vi "generate_DAC_voltages.vi"(8 "derived values":T1, 9 "scan specification":T4={"x amplitude"=0, "x resolution (pixels)"=0, "x offset fly-forward (iterations)"=0, "x offset fly-back (iterations)"=0, "y resolution (nr. of lines)"=0, "y step size"=0, "iterations per pixel"=0, "number of frames"=0, "y offset (pixels)"=0, "number of y-brake lines  (before y-fly-back)"=0, "number y-brake lines (after y-fly-back)"=0, "number of y-fly-back steps"=8, "lines per z step"=0, "number of z/intensity tuples"=0}, 10 "counter cluster in":T2, 11 "resonant trigger":bool) -> (0 "acquire?":bool, 1 "fly-back acquisition phase?":bool, 2 "counter cluster out":T2, 3 "DAC voltages":T3 {"z-drive out" max=4095 step=1; "ch6" max=4095 step=1; "ch5" max=4095 step=1; "ch4" max=4095 step=1; "ch3" max=4095 step=1; "ch2" max=4095 step=1; "ch1" max=4095 step=1; "ch0" max=4095 step=1})   [LabVIEW 2010]
uses:
  scan_specification_cluster.ctl
  common_typedefs/DAC_voltage_cluster.ctl
  counter_cluster.ctl
  derived_values_cluster.ctl
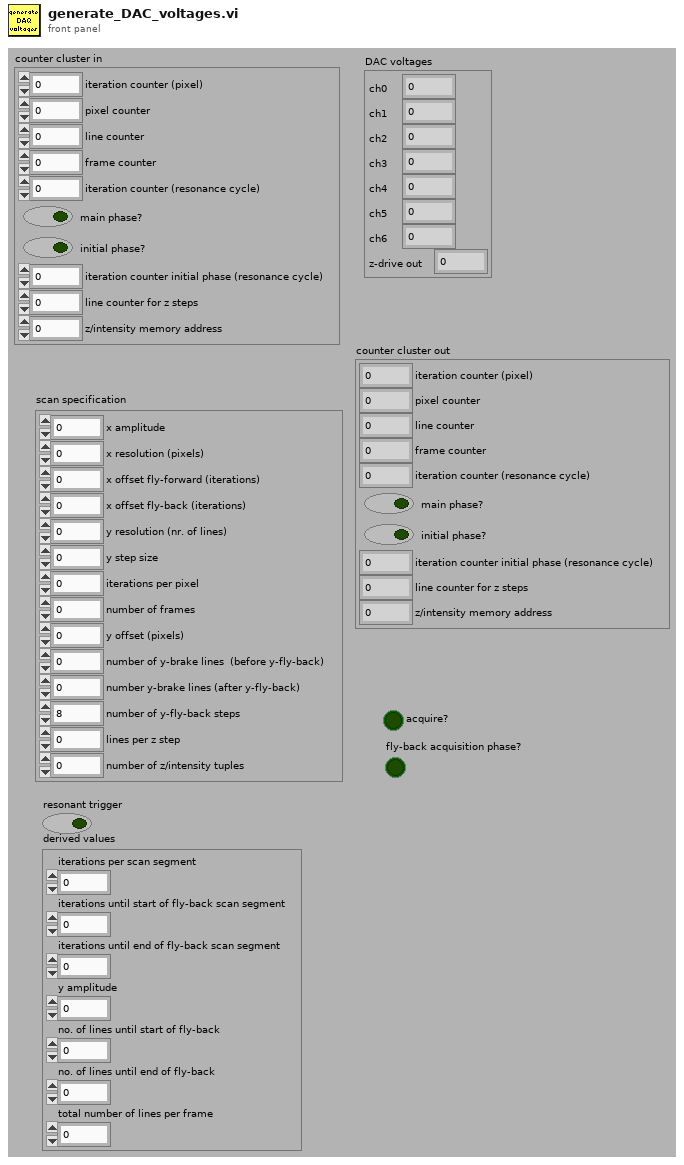
[diagram p1: front panel]
types:
  T1 = typedef "derived_values_cluster.ctl" = cluster{"iterations per scan segment":u16, "iterations until start of fly-back scan segment":u16, "iterations until end of fly-back scan segment":u16, "y amplitude":u16, "no. of lines until start of fly-back":u16, "no. of lines until end of fly-back":u16, "total number of lines per frame ":u16}
  T2 = typedef "counter_cluster.ctl" = cluster{"iteration counter (pixel)":u16, "pixel counter":u16, "line counter":u16, "frame counter":u16, "iteration counter (resonance cycle)":u16, "main phase?":bool, "initial phase?":bool, "iteration counter initial phase (resonance cycle)":u16, "line counter for z steps":u16, "z/intensity memory address":u32}
  T3 = typedef "DAC_voltage_cluster.ctl" = cluster{"ch0":u16, "ch1":u16, "ch2":u16, "ch3":u16, "ch4":u16, "ch5":u16, "ch6":u16, "z-drive out":u16}
  T4 = typedef "scan_specification_cluster.ctl" = cluster{"x amplitude":u16, "x resolution (pixels)":u16, "x offset fly-forward (iterations)":u16, "x offset fly-back (iterations)":u16, "y resolution (nr. of lines)":u16, "y step size":u16, "iterations per pixel":u16, "number of frames":i32, "y offset (pixels)":u16, "number of y-brake lines  (before y-fly-back)":u16, "number y-brake lines (after y-fly-back)":u16, "number of y-fly-back steps":u16, "lines per z step":u16, "number of z/intensity tuples":u16}
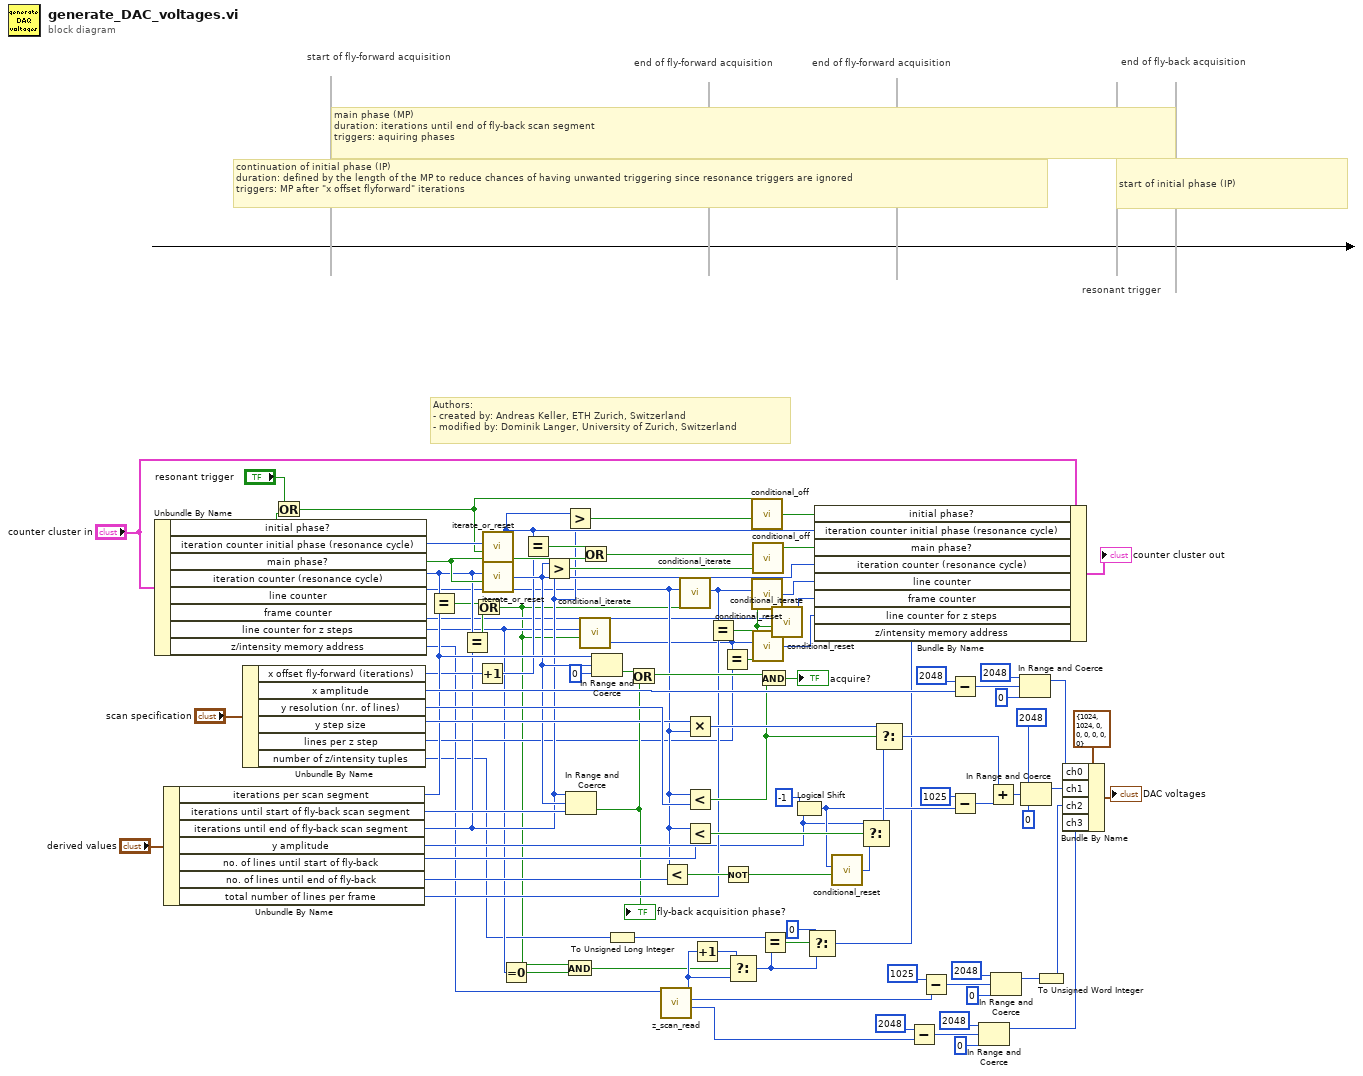
[diagram p0: block diagram]
diagram:
  # "start of initial phase (IP)"
  # "continuation of initial phase (IP)\nduration: defined by the length of the MP to reduce chances of having unwanted triggering since resonance triggers are ignored\ntriggers: MP after \"x offset flyforward\" iterations"
  # "end of fly-back acquisition"
  # "end of fly-forward acquisition"
  # "end of fly-forward acquisition"
  # "start of fly-forward acquisition"
  # "main phase (MP)\nduration: iterations until end of fly-back scan segment\ntriggers: aquiring phases"
  # "resonant trigger"
  # "Authors: \n- created by: Andreas Keller, ETH Zurich, Switzerland\n- modified by: Dominik Langer, University of Zurich, Switzerland"
  n1 = Unbundle By Name("counter cluster in") -> ("initial phase?"=w64:bool, "iteration counter initial phase (resonance cycle)"=w58:u16, "main phase?"=w57:bool, "iteration counter (resonance cycle)"=w39:u16, "line counter"=w36:u16, "frame counter"=w31:u16, "line counter for z steps"=w26:u16, "z/intensity memory address"=w25:u32)
  n2 = Unbundle By Name("derived values") -> ("iterations per scan segment"=w61:u16, "iterations until start of fly-back scan segment"=w66:u16, "iterations until end of fly-back scan segment"=w38:u16, "y amplitude"=w46:u16, "no. of lines until start of fly-back"=w45:u16, "no. of lines until end of fly-back"=w65:u16, "total number of lines per frame"=w62:u16)
  n3 = Unbundle By Name("scan specification") -> ("x offset fly-forward (iterations)"=w43:u16, "x amplitude"=w75:u16, "y resolution (nr. of lines)"=w72:u16, "y step size"=w71:u16, "lines per z step"=w32:u16, "number of z/intensity tuples"=w22:u16)
  n4 = Or(x="resonant trigger", y=w64) -> (x .or. y?=w54:bool)
  n5 = Equal?(x=w39, y=w61) -> (x = y?=w33:bool)
  n6 = Equal?(x=w39, y=w38) -> (x = y?=w37:bool)
  n7 = Or(x=w33, y=w37) -> (x .or. y?=w2:bool)
  n8 = Increment(x=w43) -> (x+1=w42:u16)
  n9 = call "iterate_or_reset.vi"("iterate?"=w54, "number in"=w58) -> ("number out"=w40:u16)  [unwired: 4 in]
  n10 = call "iterate_or_reset.vi"("iterate?"=w57, "number in"=w39) -> ("number out"=w56:u16)  [unwired: 4 in]
  n11 = Equal To 0?(x=w26) -> (x = 0?=w3:bool)
  n12 = Equal?(x=w40, y=w42) -> (x = y?=w55:bool)
  n13 = Greater?(x=w56, y=w38) -> (0:w52:bool)
  n14 = Greater?(x=w40, y=w38) -> (0:w41:bool)
  n15 = And(x=w2, y=w3) -> (x .and. y?=w1:bool)
  n16 = In Range and Coerce(upper limit=w38, x=w56, lower limit=w66) -> (In Range?=w34:bool)  [unwired: 1 out]
  "fly-back acquisition phase?" <- w34
  n17 = call "conditional_iterate.vi"("iterate?"=w2, "number in"=w26) -> ("number out"=w27:u16)  [unwired: 4 in]
  n18 = Or(x=w55, y=w57) -> (x .or. y?=w51:bool)
  n19 = In Range and Coerce(upper limit=w61, x=w56, lower limit=u16 0) -> (In Range?=w87:bool)  [unwired: 1 out]
  n20 = To Unsigned Long Integer(number=w22) -> (unsigned 32bit integer=w21:u32)
  n21 = Or(x=w87, y=w34) -> (x .or. y?=w70:bool)
  n22 = call "z_scan_read.vi"("address in"=w25) -> ("intensity"=w12:u16, "z-value"=w5:i16, "address out"=w24:u32)  [unwired: 8 in]
  n23 = Less?(x=w36, y=w65) -> (x < y?=w68:bool)
  n24 = call "conditional_iterate.vi"("iterate?"=w2, "number in"=w36) -> ("number out"=w35:u16)  [unwired: 4 in]
  n25 = Multiply(x=w71, y=w36) -> (x*y=w93:u16)
  n26 = Less?(x=w36, y=w72) -> (x < y?=w69:bool)
  n27 = Less?(x=w36, y=w45) -> (x < y?=w95:bool)
  n28 = Increment(x=w24) -> (x+1=w23:u32)
  n29 = Equal?(x=w35, y=w62) -> (x = y?=w44:bool)
  n30 = Equal?(x=w27, y=w32) -> (x = y?=w28:bool)
  n31 = Not(x=w68) -> (.not. x?=w48:bool)
  n32 = Select(t=w23, s=w1, f=w24) -> (s? t:f=w18:u32)
  n33 = call "conditional_off.vi"("switch off?"=w41, "boolean in"=w54) -> ("boolean out"=w53:bool)  [unwired: 4 in]
  n34 = call "conditional_reset.vi"("reset?"=w44, "number in"=w35) -> ("number out"=w59:u16)  [unwired: 4 in]
  n35 = call "conditional_off.vi"("switch off?"=w52, "boolean in"=w51) -> ("boolean out"=w50:bool)  [unwired: 4 in]
  n36 = call "conditional_reset.vi"("reset?"=w28, "number in"=w27) -> ("number out"=w29:u16)  [unwired: 4 in]
  n37 = And(x=w70, y=w69) -> (x .and. y?=→"acquire?":bool)
  n38 = Equal?(x=w21, y=w18) -> (x = y?=w20:bool)
  n39 = call "conditional_iterate.vi"("iterate?"=w44, "number in"=w31) -> ("number out"=w30:u16)  [unwired: 4 in]
  n40 = Logical Shift(y=i16 -1 ("n"), x=w46) -> (x << y=w49:u16)
  n41 = Select(t=u32 0, s=w20, f=w18) -> (s? t:f=w19:u32)
  n42 = Bundle By Name(cluster="counter cluster in", "initial phase?"=w53, "iteration counter initial phase (resonance cycle)"=w40, "main phase?"=w50, "iteration counter (resonance cycle)"=w56, "line counter"=w59, "frame counter"=w30, "line counter for z steps"=w29, "z/intensity memory address"=w19) -> (→"counter cluster out":T2)
  n43 = call "conditional_reset.vi"("reset?"=w48, "number in"=w49) -> ("number out"=w47:u16)  [unwired: 4 in]
  n44 = Select(t=w46, s=w95, f=w47) -> (s? t:f=w94:u16)
  n45 = Select(t=w93, s=w69, f=w94) -> (s? t:f=w73:u16)
  n46 = Subtract(x=u16 2048, y=w12) -> (x-y=w14:u16)
  n47 = Subtract(x=i16 1025, y=w5) -> (x-y=w9:i16)
  n48 = Subtract(x=u16 2048, y=w75) -> (x-y=w79:u16)
  n49 = Subtract(x=u16 1025, y=w49) -> (x-y=w86:u16)
  n50 = In Range and Coerce(upper limit=u16 2048, x=w14, lower limit=u16 0) -> (coerced(x)=w11:u16)  [unwired: 1 out]
  n51 = Add(x=w73, y=w86) -> (x+y=w82:u16)
  n52 = In Range and Coerce(upper limit=i16 2048, x=w9, lower limit=i16 0) -> (coerced(x)=w6:i16)  [unwired: 1 out]
  n53 = In Range and Coerce(upper limit=u16 2048, x=w79, lower limit=u16 0) -> (coerced(x)=w78:u16)  [unwired: 1 out]
  n54 = In Range and Coerce(upper limit=u16 2048, x=w82, lower limit=u16 0) -> (coerced(x)=w81:u16)  [unwired: 1 out]
  n55 = To Unsigned Word Integer(number=w6) -> (unsigned 16bit integer=w4:u16)
  n56 = Bundle By Name(cluster=T3 {"ch0"=1024, "ch1"=1024, "ch2"=0, "ch3"=0, "ch4"=0, "ch5"=0, "ch6"=0, "z-drive out"=0} ("DAC voltage"), "ch0"=w78, "ch1"=w81, "ch2"=w4, "ch3"=w11) -> (→"DAC voltages":T3)
